vi "PlayMediaPlayerFile.vi"(6 "Size":string(combo)="C:\\Users\\ThomasWattson\\OneDrive - Rage Systems\\Documents - Tetra\\Test Docs\\WAM ATE MEDIA\\FieldTest_RFSM-Only.mp4", 11 "path":path) -> ()   [LabVIEW 2018]
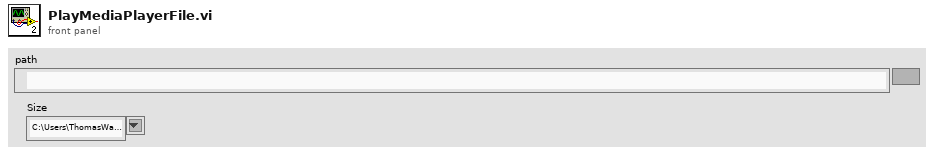
[diagram p1: front panel]
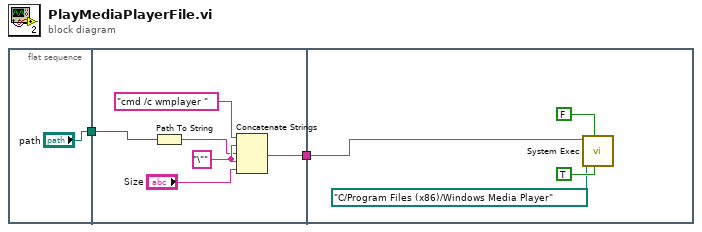
[diagram p0: block diagram]
diagram:
  n1 = flat-sequence {
    tunnel: ["path"] -> w2
    tunnel: w2 -> [w5]
    tunnel: [w8] -> w1
    tunnel: w1 -> [w10]
    frame #0 {
    }
    frame #1 {
      w7 = "\""
      n2 = Path To String(path=w5) -> (string=w6:string)
      n3 = Concatenate Strings("cmd /c wmplayer " ("command line"), w7, w6, w7, "Size") -> (w8:string)
    }
    frame #2 {
      n4 = call <vilib>:"System Exec.vi"("run minimized? (F)"=TRUE, "wait until completion? (T)"=FALSE, "working directory"=path "C:/Program Files (x86)/Windows Media Player", "command line"=w10) -> ()  [unwired: 4 in, 4 out]
    }
  }
